vi "_unstackArray.vi"(11 "Stacked Array":dbl[](array[numeric])) -> (2 "Inner dimensions":dbl[][](array[numeric]), 3 "Unstacked Array":dbl[][][](array[numeric]))   [LabVIEW 2021, in "System.lvclass"]
uses:
  System.lvclass
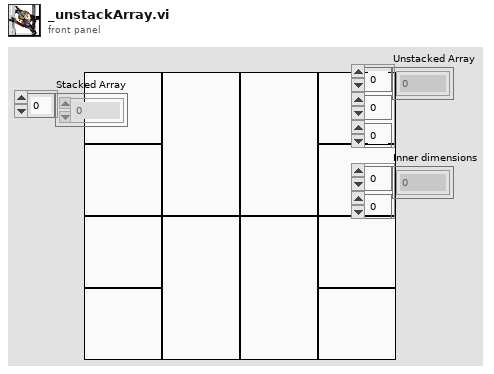
[diagram p1: front panel]
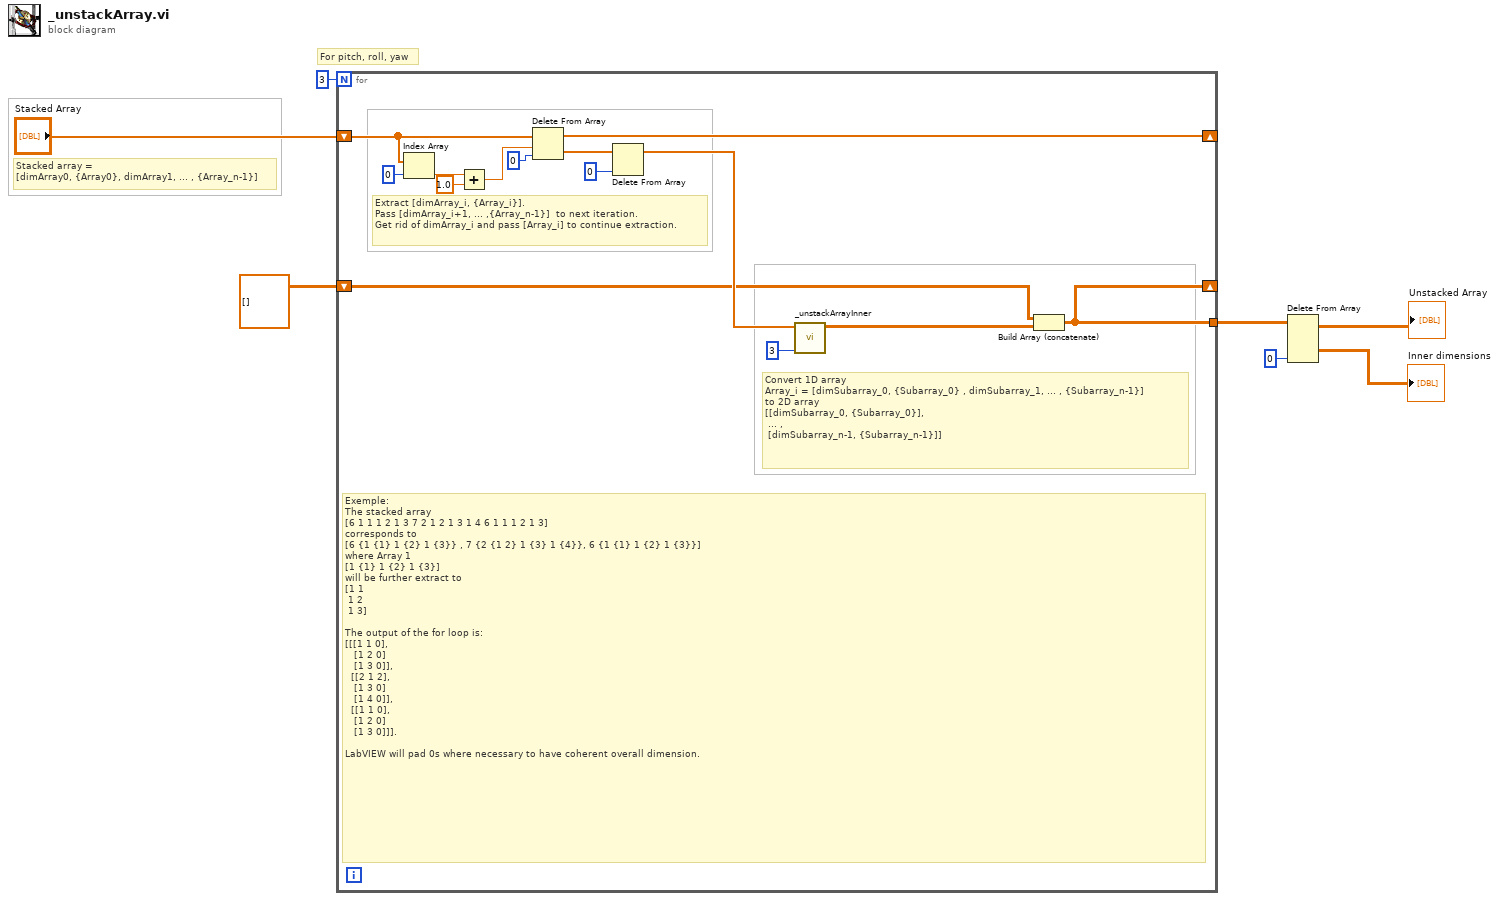
[diagram p0: block diagram]
diagram:
  # "Stacked array = \n[dimArray0, {Array0}, dimArray1, ... , {Array_n-1}]"
  # "For pitch, roll, yaw"
  n1 = for {
    N: 3 -> [_]
    shift-right: [w18] -> _
    shift-left: "Stacked Array" -> [w19]
    shift-right: [w10] -> _
    shift-left: dbl[][][] [] -> [w12]
    tunnel: [w10] -> w5
    # "Exemple:\nThe stacked array\n[6 1 1 1 2 1 3 7 2 1 2 1 3 1 4 6 1 1 1 2 1 3]\ncorresponds to\n[6 {1 {1} 1 {2} 1 {3}} , 7 {2 {1 2} 1 {3} 1 {4}}, 6 {1 {1} 1 {2} 1 {3}}]\nwhere Array 1\n[1 {1} 1 {2} 1 {3}]\nwill be further extract to \n[1 1 \n 1 2\n 1 3]\n\nThe output of the for loop is:\n[[[1 1 0],\n   [1 2 0]\n   [1 3 0]],\n  [[2 1 2],\n   [1 3 0]\n   [1 4 0]],\n  [[1 1 0],\n   [1 2 0]\n   [1 3 0]]].\n\nLabVIEW will pad 0s where necessary to have coherent overall dimension."
    # "Convert 1D array\nArray_i = [dimSubarray_0, {Subarray_0} , dimSubarray_1, ... , {Subarray_n-1}]\nto 2D array \n[[dimSubarray_0, {Subarray_0}], \n ... ,\n [dimSubarray_n-1, {Subarray_n-1}]]"
    # "Extract [dimArray_i, {Array_i}].\nPass [dimArray_i+1, ... ,{Array_n-1}]  to next iteration.\nGet rid of dimArray_i and pass [Array_i] to continue extraction."
    n2 = Index Array(array=w19, index=0) -> (element=w17:dbl)
    n3 = Add(x=w17, y=1.0) -> (x+y=w8:dbl)
    n4 = Delete From Array(array=w19, length=w8, index=0) -> (deleted portion=w15:dbl[], array with subset deleted=w18:dbl[])
    n5 = Delete From Array(array=w15, index=0) -> (array with subset deleted=w13:dbl[])  [unwired: 1 in, 1 out]
    n6 = call "_unstackArrayInner.vi"("#iter"=3, "Stacked Array"=w13) -> ("Unstacked Array"=w11:dbl[][])  [unwired: 9 in]
    n7 = Build Array (concatenate)(w12, w11) -> (w10:dbl[][][])
  }
  n8 = Delete From Array(array=w5, index (dim 2)=0 ("disabled index (col)")) -> (deleted portion=→"Inner dimensions":dbl[][], array with subset deleted=→"Unstacked Array":dbl[][][])  [unwired: 3 in]
